vi "Lockin and Keithley Multimeter.vi"(8 "error in (no error)":errorcluster, 11 "Lockin and Keithley Multimeter in":refnum<class "Lockin and Keithley Multimeter.lvclass">) -> (0 "error out":errorcluster, 3 "Lockin and Keithley Multimeter out":refnum<class "Lockin and Keithley Multimeter.lvclass">)   [LabVIEW 2017, in "Lockin and Keithley Multimeter.lvclass"]
uses:
  Lockin and Keithley Multimeter.lvclass
  C:/LabVIEW-programs/Instruments/Utility Classes/Readable/Readable.lvclass
  Lockin and Keithley Multimeter.lvclass/Lockin and Keithley Multimeter.ctl
  Global/GPIB Numbers.vi
  Utility Classes/Readable/Readable.lvclass
panel:
  out "Status":string
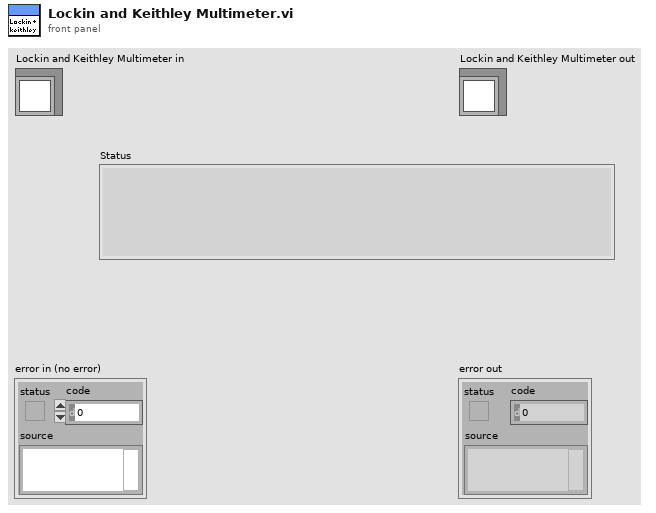
[diagram p1: front panel]
types:
  T1 = typedef "GPIB Type Def.ctl" = cluster{"Name":string, "bus":dbl, "GPIB":dbl, "GPIB as string":string, "byte":i32, "VISA Resource Name":refnum<visa-resource-name>}
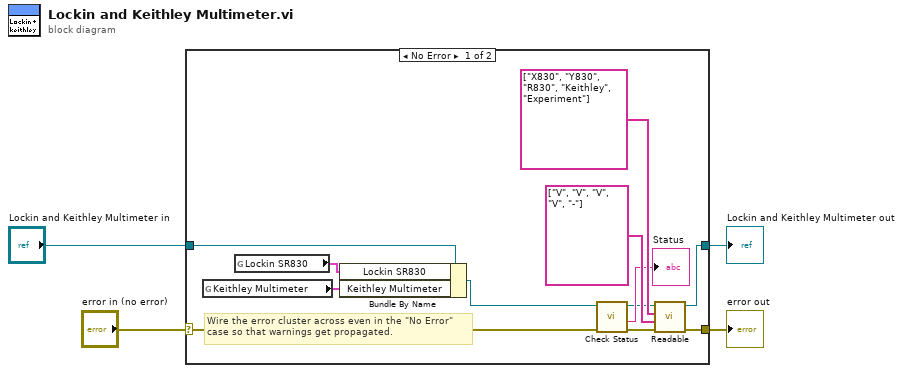
[diagram p0: block diagram]
diagram:
  n1 = case shown="No Error" "error in (no error)" {
    selector: "error in (no error)" -> [w12 w18]
    tunnel: [w8 w18] -> w3
    tunnel: [w5 w17] -> w1
    tunnel: "Lockin and Keithley Multimeter in" -> [w14 w17]
    frame No Error {
      # "Wire the error cluster across even in the \"No Error\"\ncase so that warnings get propagated."
      n2 = global read "GPIB Numbers.vi" "Keithley Multimeter"() -> (w15:T1)
      n3 = global read "GPIB Numbers.vi" "Lockin SR830"() -> (w16:T1)
      n4 = Bundle By Name(cluster=w14, "Lockin SR830"=w16, "Keithley Multimeter"=w15) -> (w13:refnum<class "Lockin and Keithley Multimeter.lvclass">)
      n5 = call-dynamic "Check Status.vi"("error in (no error)"=w12, "Lockin and Keithley Multimeter in"=w13) -> ("error out"=w9:errorcluster, "Status"=→"Status":string, "Lockin and Keithley Multimeter out"=w6:refnum<class "Lockin and Keithley Multimeter.lvclass">)  [unwired: 6 in, 1 out]
      n6 = call "Readable.vi"("error in (no error)"=w9, "Channel Units"=string[] ["V", "V", "V", "V", "-"], "Channel Names"=string[] ["X830", "Y830", "R830", "Keithley", "Experiment"], "Readable in"=w6) -> ("error out"=w8:errorcluster, "Readable out"=w5:refnum<class "Lockin and Keithley Multimeter.lvclass">)  [unwired: 6 in]
    }
    frame Error {
    }
  }
  "error out" <- w3
  "Lockin and Keithley Multimeter out" <- w1
